vi "MPExxx Error Query.vi"(0 "VISA session":refnum<visa-resource-name>, 1 "error in (no error)":errorcluster {"code" format="%.0x"}) -> (2 "dup VISA session":refnum<visa-resource-name>, 3 "Error":i32, 4 "Error Message":string, 5 "error out":errorcluster {"code" format="%.0x"})   [LabVIEW 2012]
doc: "This VI reads an error from the instrument. It expects to see errors in SCPI format (#,\"error message\"). If an error query is not supported, it returns a warning."
panel:
  # "MAGNA-POWER"
  # "Electronics"
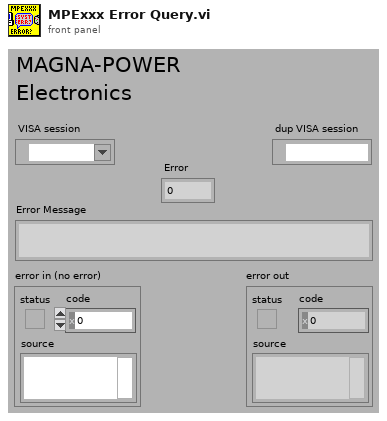
[diagram p1: front panel]
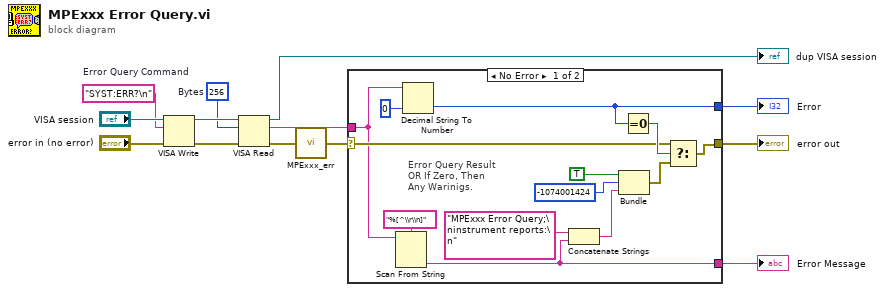
[diagram p0: block diagram]
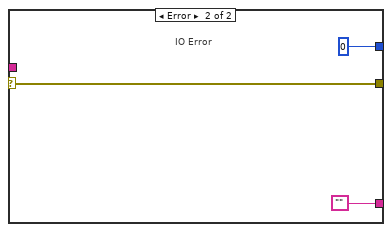
[diagram p2: hidden frame]
diagram:
  w6 = u32 256  # Bytes
  w4 = "SYST:ERR?\n"  # Error Query Command
  n1 = VISA Write(VISA resource name="VISA session", write buffer=w4, error in (no error)="error in (no error)") -> (VISA resource name out=w7:refnum<visa-resource-name>, error out=w5:errorcluster)  [unwired: 1 out]
  n2 = VISA Read(VISA resource name=w7, byte count=w6, error in (no error)=w5) -> (VISA resource name out=→"dup VISA session":refnum<visa-resource-name>, read buffer=w3:string, error out=w2:errorcluster)  [unwired: 1 out]
  n3 = call "MPExxx_err.vi"("error in (no error)"=w2) -> ("error out"=w1:errorcluster)
  n4 = case shown="No Error" w1 {
    selector: w1 -> [w17 w27]
    tunnel: w3 -> [w15 _]
    tunnel: [w22 w27] -> w8
    tunnel: [w18 ""] -> w13
    tunnel: [w14 0] -> w12
    frame No Error {
      # "Error Query Result\nOR If Zero, Then\nAny Warinigs."
      n5 = Scan From String(format string="%[^\\r\\n]", input string=w15) -> (output 1=w18:string)  [unwired: 3 in, 3 out]
      n6 = Decimal String To Number(string=w15, default (0L)=0) -> (number=w14:i32)  [unwired: 1 in, 1 out]
      n7 = Concatenate Strings("MPExxx Error Query;\ninstrument reports:\n" ("Source"), w18) -> (w24:string)
      n8 = Bundle("Status"=TRUE, "Code"=-1074001424, w24) -> (w23:cluster{"Status":bool, "Code":i32, string})  [unwired: 1 in]
      n9 = Equal To 0?(x=w14) -> (x = 0?=w20:bool)
      n10 = Select(t=w17, s=w20, f=w23) -> (s? t:f=w22:errorcluster)
    }
    frame Error {
      # "IO Error"
    }
  }
  "Error Message" <- w13
  "Error" <- w12
  "error out" <- w8
